vi "Counter.vi"() -> (3 "Numeric":u64)   [LabVIEW 2018]
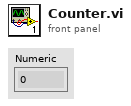
[diagram p1: front panel]
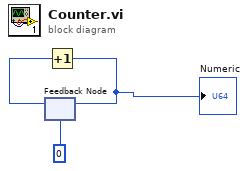
[diagram p0: block diagram]
diagram:
  n1 = feedback #1(i16 0) -> (w2:i16)
  n2 = Increment(x=w2) -> (x+1=w3:i16)
  "Numeric" <- w3
  n3 = feedback-in #1(w3) -> ()
